vi "VisionAnalysis.vi"(0 "Image In":T1, 7 "error in":errorcluster) -> (20 "Image Out":T1, 21 "Number of Particles (Particle Analysis 1)":i32, 22 "Particle Measurements (Pixels) (Particle Analysis 1)":dbl[][](array[numeric]) format="%.2f", 27 "error out":errorcluster)   [LabVIEW 2015]
uses:
  <vilib>/vision/Image Controls.llb/IMAQ Image.ctl
  <vilib>/vision/NI_Vision_Development_Module.lvlib
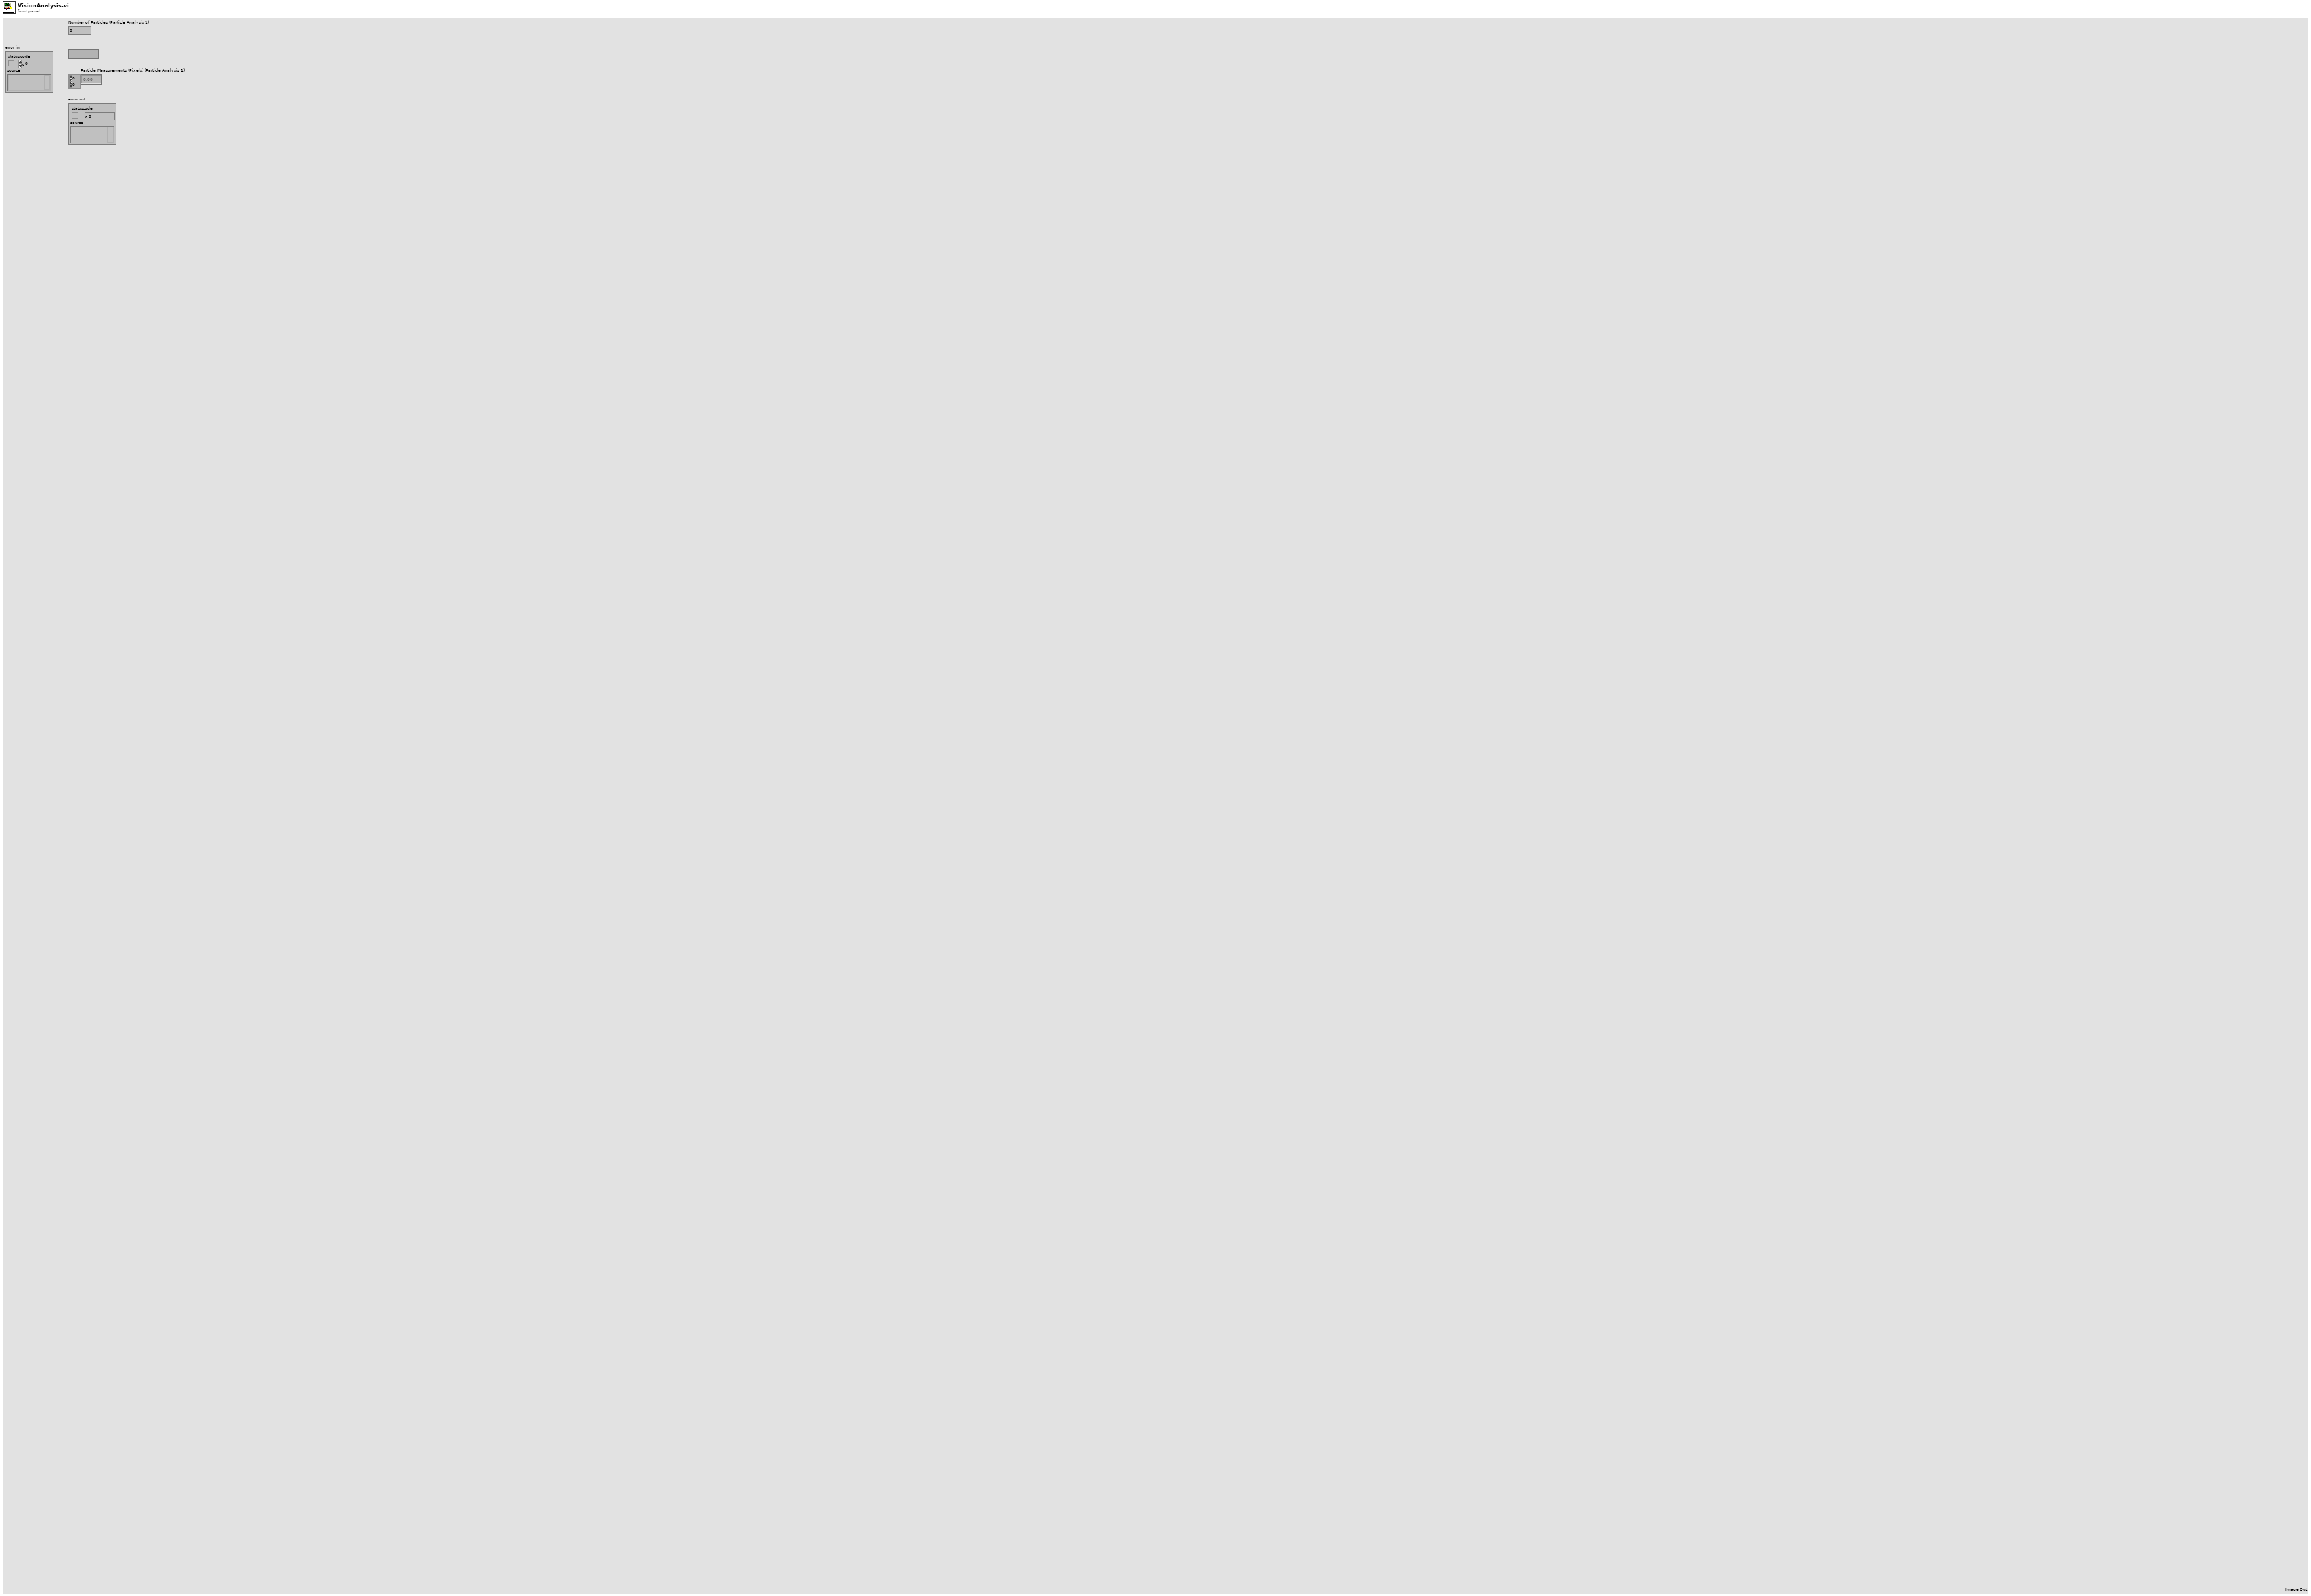
[diagram p1: front panel]
types:
  T1 = typedef "IMAQ Image.ctl" = refnum<image>
  T2 = cluster{"Measurement Parameter":i32, "Range Lower Value":dbl, "Range Upper Value":dbl, "Range":bool, "Measurement Type":bool}[]
  T3 = enum32{"AutoM", "Close", "Dilate", "Erode", "Gradient", "Gradient out", "Gradient in", "Hit miss", "Open", "PClose", "POpen", "Thick", "Thin"}
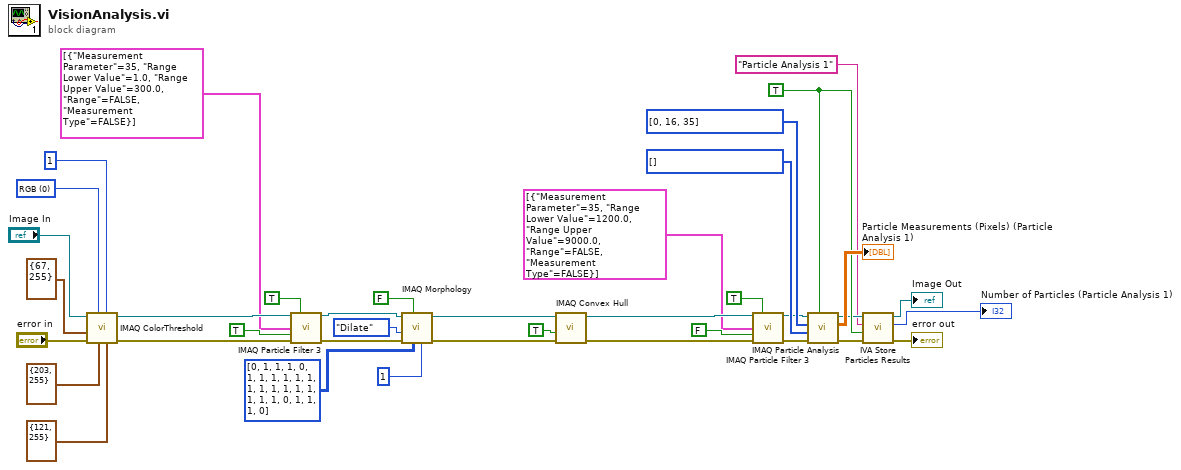
[diagram p0: block diagram]
diagram:
  w11 = i32[] [] items=["Center of Mass X", "Center of Mass Y", "First Pixel X", "First Pixel Y", "Bounding Rect Left", "Bounding Rect Top", "Bounding Rect Right", "Bounding Rect Bottom", "Max Feret Diameter Start X", "Max Feret Diameter Start Y", "Max Feret Diameter End X", "Max Feret Diameter End Y", "Max Horiz. Segment Length Left", "Max Horiz. Segment Length Right", "Max Horiz. Segment Length Row", "-", "Bounding Rect Width", "Bounding Rect Height", "Bounding Rect Diagonal", "Perimeter", "Convex Hull Perimeter", "Holes' Perimeter", "Max Feret Diameter", "Equivalent Ellipse Major Axis", "Equivalent Ellipse Minor Axis", "Equivalent Ellipse Minor Axis (Feret)", "Equivalent Rect Long Side", "Equivalent Rect Short Side", "Equivalent Rect Diagonal", "Equivalent Rect Short Side (Feret)", "Average Horiz. Segment Length", "Average Vert. Segment Length", "Hydraulic Radius", "Waddel Disk Diameter", "-", "Area", "Holes' Area", "Particle & Holes' Area", "Convex Hull Area", "Image Area", "-", "Number of Holes", "Number of Horiz. Segments", "Number of Vert. Segments", "-", "Orientation", "Max Feret Diameter Orientation", "-", "% Area/Image Area", "% Area/(Particle & Holes' Area)", "Ratio of Equivalent Ellipse Axes", "Ratio of Equivalent Rect Sides", "-", "Elongation Factor", "Compactness Factor", "Heywood Circularity Factor", "Type Factor", "-", "Sum X", "Sum Y", "Sum XX", "Sum XY", "Sum YY", "Sum XXX", "Sum XXY", "Sum XYY", "Sum YYY", "-", "Moment of Inertia XX", "Moment of Inertia XY", "Moment of Inertia YY", "Moment of Inertia XXX", "Moment of Inertia XXY", "Moment of Inertia XYY", "Moment of Inertia YYY", "Norm. Moment of Inertia XX", "Norm. Moment of Inertia XY", "Norm. Moment of Inertia YY", "Norm. Moment of Inertia XXX", "Norm. Moment of Inertia XXY", "Norm. Moment of Inertia XYY", "Norm. Moment of Inertia YYY", "Hu Moment 1", "Hu Moment 2", "Hu Moment 3", "Hu Moment 4", "Hu Moment 5", "Hu Moment 6", "Hu Moment 7"] ("Real-World Measurements")
  w12 = i32[] [0, 16, 35] items=["Center of Mass X", "Center of Mass Y", "First Pixel X", "First Pixel Y", "Bounding Rect Left", "Bounding Rect Top", "Bounding Rect Right", "Bounding Rect Bottom", "Max Feret Diameter Start X", "Max Feret Diameter Start Y", "Max Feret Diameter End X", "Max Feret Diameter End Y", "Max Horiz. Segment Length Left", "Max Horiz. Segment Length Right", "Max Horiz. Segment Length Row", "-", "Bounding Rect Width", "Bounding Rect Height", "Bounding Rect Diagonal", "Perimeter", "Convex Hull Perimeter", "Holes' Perimeter", "Max Feret Diameter", "Equivalent Ellipse Major Axis", "Equivalent Ellipse Minor Axis", "Equivalent Ellipse Minor Axis (Feret)", "Equivalent Rect Long Side", "Equivalent Rect Short Side", "Equivalent Rect Diagonal", "Equivalent Rect Short Side (Feret)", "Average Horiz. Segment Length", "Average Vert. Segment Length", "Hydraulic Radius", "Waddel Disk Diameter", "-", "Area", "Holes' Area", "Particle & Holes' Area", "Convex Hull Area", "Image Area", "-", "Number of Holes", "Number of Horiz. Segments", "Number of Vert. Segments", "-", "Orientation", "Max Feret Diameter Orientation", "-", "% Area/Image Area", "% Area/(Particle & Holes' Area)", "Ratio of Equivalent Ellipse Axes", "Ratio of Equivalent Rect Sides", "-", "Elongation Factor", "Compactness Factor", "Heywood Circularity Factor", "Type Factor", "-", "Sum X", "Sum Y", "Sum XX", "Sum XY", "Sum YY", "Sum XXX", "Sum XXY", "Sum XYY", "Sum YYY", "-", "Moment of Inertia XX", "Moment of Inertia XY", "Moment of Inertia YY", "Moment of Inertia XXX", "Moment of Inertia XXY", "Moment of Inertia XYY", "Moment of Inertia YYY", "Norm. Moment of Inertia XX", "Norm. Moment of Inertia XY", "Norm. Moment of Inertia YY", "Norm. Moment of Inertia XXX", "Norm. Moment of Inertia XXY", "Norm. Moment of Inertia XYY", "Norm. Moment of Inertia YYY", "Hu Moment 1", "Hu Moment 2", "Hu Moment 3", "Hu Moment 4", "Hu Moment 5", "Hu Moment 6", "Hu Moment 7"] ("Pixel Measurements")
  w7 = TRUE ("Connectivity 4/8 (8)")
  w37 = u16 0 items=["RGB", "HSL", "HSV", "HSI"] ("Color Mode")
  n1 = call "IMAQ ColorThreshold"("Blue or Luma or Val or Inten Range"=cluster{"Lower value":i32, "Upper value":i32} {"Lower value"=121, "Upper value"=255}, "Replace Value"=1, "Green or Sat Range"=cluster{"Lower value":i32, "Upper value":i32} {"Lower value"=203, "Upper value"=255}, "Color Mode"=w37, "error in (no error)"="error in", "Red or Hue Range"=cluster{"Lower value":i32, "Upper value":i32} {"Lower value"=67, "Upper value"=255}, "Image Src"="Image In") -> ("error out"=w28:errorcluster, "Image Dst Out"=w29:T1)  [unwired: 1 in, 2 out]
  n2 = call "IMAQ Particle Filter 3"("Image Src"=w29, "Connectivity 4/8 (8)"=TRUE, "Selection Values"=T2 [{"Measurement Parameter"=35, "Range Lower Value"=1.0, "Range Upper Value"=300.0, "Range"=FALSE, "Measurement Type"=FALSE}], "Keep/Remove Particles (F)"=TRUE ("Keep/Remove Particles"), "error in (no error)"=w28) -> ("Image Dst Out"=w22:T1, "error out"=w21:errorcluster)  [unwired: 4 in, 5 out]
  n3 = call "IMAQ Morphology"("Number of iterations (1)"=1, "Structuring Element"=i32[][] [[0, 1, 1, 1, 0], [1, 1, 1, 1, 1], [1, 1, 1, 1, 1], [1, 1, 1, 1, 1], [0, 1, 1, 1, 0]], "Square/Hexa (Square)"=FALSE, "error in (no error)"=w21, "Operation"=T3."Dilate", "Image Src"=w22) -> ("error out"=w19:errorcluster, "Image Dst Out"=w20:T1)  [unwired: 1 in, 3 out]
  n4 = call "IMAQ Convex Hull"("error in (no error)"=w19, "Connectivity 4/8 (8)"=TRUE, "Image Src"=w20) -> ("error out"=w14:errorcluster, "Image Dst Out"=w15:T1)  [unwired: 1 in, 6 out]
  n5 = call "IMAQ Particle Filter 3"("Image Src"=w15, "Connectivity 4/8 (8)"=TRUE, "Selection Values"=T2 [{"Measurement Parameter"=35, "Range Lower Value"=1200.0, "Range Upper Value"=9000.0, "Range"=FALSE, "Measurement Type"=FALSE}], "Keep/Remove Particles (F)"=FALSE ("Keep/Remove Particles"), "error in (no error)"=w14) -> ("Image Dst Out"=w8:T1, "error out"=w9:errorcluster)  [unwired: 4 in, 5 out]
  n6 = call "IMAQ Particle Analysis"("Connectivity 4/8 (8)"=w7, "error in (no error)"=w9, "Real-World Measurements"=w11, "Pixel Measurements"=w12, "Image"=w8) -> ("error out"=w3:errorcluster, "Particle Measurements (Pixels)"=→"Particle Measurements (Pixels) (Particle Analysis 1)":dbl[][], "Image Out (duplicate)"=w6:T1)  [unwired: 4 out]
  n7 = call <vilib>:"IVA Store Particles Results.vi"("error in (no error)"=w3, "Connectivity 4/8 (8)"=w7, "Step Name"="Particle Analysis 1", "Image in"=w6) -> ("error out"=→"error out":errorcluster, "Number of Particles"=→"Number of Particles (Particle Analysis 1)":i32, "Image dup"=→"Image Out":T1)  [unwired: 5 out]
